vi "Multiplexer.vi"(2 "continousSequencer?":bool, 3 "write":bool, 4 "nOfChannels":u8 format="%08b", 5 "Data":u32[](array[numeric])=[0, 0, 0, 0, 0, 0, 0, 0]) -> (0 "done":bool)   [LabVIEW 2014]
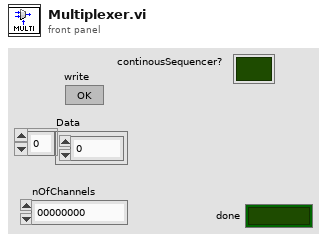
[diagram p1: front panel]
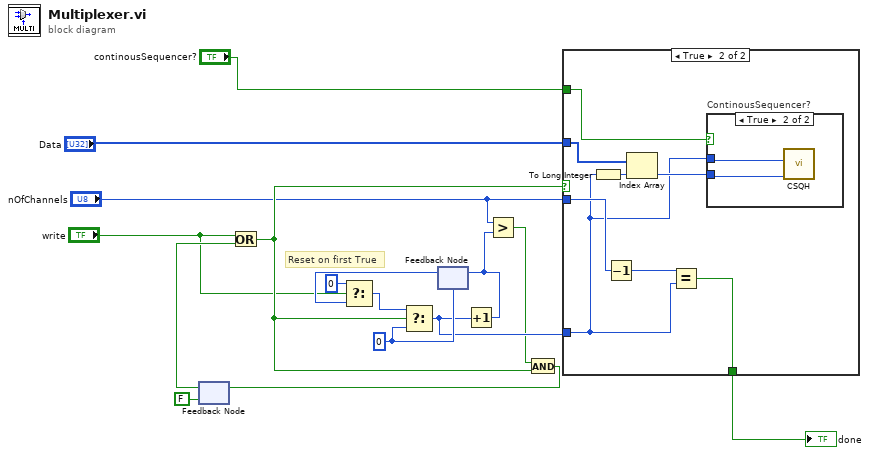
[diagram p0: block diagram]
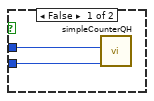
[diagram p3: hidden frame]
diagram:
  w13 = u8 0 ("nOfChannels")
  # "Reset on first True"
  n1 = feedback #1(FALSE) -> (w15:bool)
  n2 = Or(x="write", y=w15) -> (x .or. y?=w9:bool)
  n3 = feedback #2(w13) -> (w5:u8)
  n4 = Select(t=u8 0, s="write", f=w5) -> (s? t:f=w6:u8)
  n5 = Select(t=w6, s=w9, f=w13) -> (s? t:f=w12:u8)
  n6 = Increment(x=w12) -> (x+1=w11:u8)
  n7 = feedback-in #2(w11) -> ()
  n8 = Greater?(x="nOfChannels", y=w11) -> (0:w10:bool)
  n9 = And(x=w10, y=w9) -> (x .and. y?=w8:bool)
  n10 = feedback-in #1(w8) -> ()
  n11 = case shown="True" w9 {
    tunnel: "Data" -> [_ w24]
    tunnel: w12 -> [_ w19]
    tunnel: "nOfChannels" -> [_ w21]
    tunnel: [_ w18] -> w2
    tunnel: "continousSequencer?" -> [_ w17]
    frame False {
    }
    frame True {
      n12 = To Long Integer(number=w19) -> (32bit integer=w23:i32)
      n13 = Decrement(x=w21) -> (x-1=w20:u8)
      n14 = Index Array(array=w24, index=w23) -> (element=w22:u32)
      n15 = Equal?(x=w20, y=w19) -> (x = y?=w18:bool)
      n16 = case "ContinousSequencer?" shown="True" w17 {
        tunnel: w22 -> [w26 w27]
        tunnel: w19 -> [w25 w28]
        frame False {
          n17 = call "simpleCounterQH.vi"("CounterEntry"=w26, "whichPMT?"=w25) -> ()  [unwired: 9 in, 1 out]
        }
        frame True {
          n18 = call "CSQH.vi"("CounterEntry"=w27, "whichPMT?"=w28) -> ()  [unwired: 9 in, 1 out]
        }
      }
    }
  }
  "done" <- w2
